vi "_IP Reporter.vi"(4 "ignore Gateway IP?(T)":bool=TRUE, 8 "error in":errorcluster, 9 "notifier":refnum<notifier>, 10 "Init-Information":string, 11 "Setttings":T1={"address"="234.5.6.7", "receiver port"=58432, "Ignore Gateway IP"=TRUE, "HostName"=""}) -> (0 "error out":errorcluster)   [LabVIEW 2017]
doc: "Creates a write-only UDP multicast session and sends data to the specified port."
uses:
  _Typedef/Def-IniSettings -- Cluster.ctl
  _Typedef/Def-Report -- Cluster.ctl
  <vilib>/Utility/tcp.llb/UDP Multicast Write-Only Open.vi
panel:
  out "JSON string":string
  in  "Stop":bool
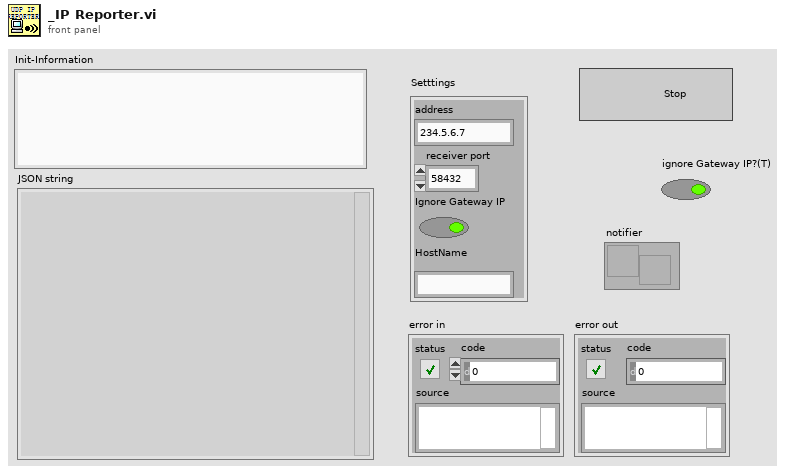
[diagram p1: front panel]
types:
  T1 = typedef "Def-IniSettings -- Cluster.ctl" = cluster{"address":string, "receiver port":u16, "Ignore Gateway IP":bool, "HostName":string}
  T2 = typedef "Def-Report -- Cluster.ctl" = cluster{"Host Name":string, "IPs":string[], "Timestamp":string, "Information":string}
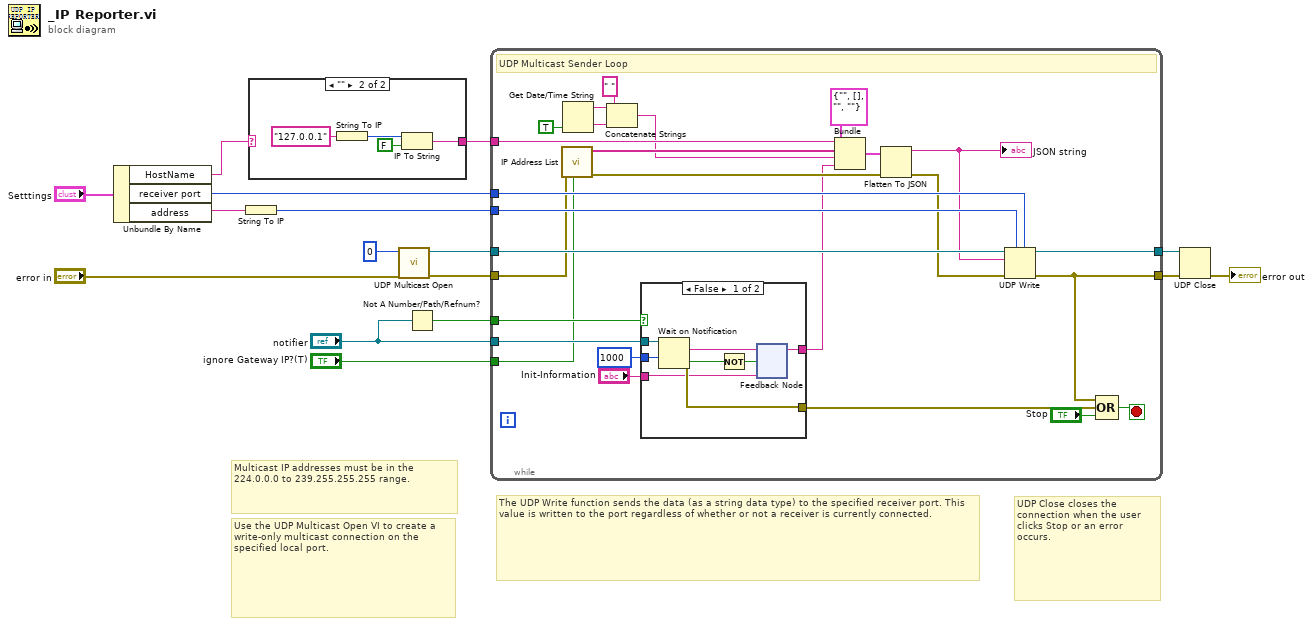
[diagram p0: block diagram]
diagram:
  # "UDP Close closes the connection when the user clicks Stop or an error occurs."
  # "Multicast IP addresses must be in the 224.0.0.0 to 239.255.255.255 range."
  # "The UDP Write function sends the data (as a string data type) to the specified receiver port. This value is written to the port regardless of whether or not a receiver is currently connected."
  # "Use the UDP Multicast Open VI to create a write-only multicast connection on the specified local port."
  n1 = Unbundle By Name("Setttings") -> ("HostName"=w8:string, "receiver port"=w10:u16, "address"=w11:string)
  n2 = String To IP(1:w11) -> (0:w14:u32)
  n3 = case shown="\"\"" w8 {
    selector: w8 -> [w17 _]
    tunnel: [w17 w21] -> w9
    frame "False", Default {
    }
    frame "" {
      n4 = String To IP(1:"127.0.0.1" ("name")) -> (0:w20:u32)
      n5 = IP To String(1:FALSE ("dot notation? (F)"), 2:w20) -> (0:w21:string)
    }
  }
  n6 = call-poly <vilib>:"UDP Multicast Open.vi"("error in (no error)"="error in", "port"=u16 0) -> ("error out"=w12:errorcluster, "connection ID"=w13:refnum<k16>)  [unwired: 8 in]
  n7 = Not A Number/Path/Refnum?(number/path/refnum="notifier") -> (NaN/Path/Refnum?=w6:bool)
  n8 = while {
    tunnel: [w30] -> w15
    tunnel: w13 -> [w48]
    tunnel: w12 -> [w42]
    tunnel: [w45] -> w16
    tunnel: w14 -> [w44]
    tunnel: w10 -> [w43]
    tunnel: w9 -> [w35]
    tunnel: "notifier" -> [w34]
    tunnel: w6 -> [w31]
    tunnel: "ignore Gateway IP?(T)" -> [w24]
    stop <- w47 stop-if-true
    # "UDP Multicast Sender Loop"
    n9 = call "IP Address List.vi"("ignore Gateway IP?"=w24, "error in (no error)"=w42) -> ("error out"=w41:errorcluster, "Array"=w37:string[])  [unwired: 8 in]
    n10 = Get Date/Time String(want seconds? (F)=TRUE) -> (date string=w29:string, time string=w28:string)  [unwired: 2 in]
    n11 = Concatenate Strings(w29, " " ("string"), w28) -> (w26:string)
    n12 = case shown="False" w31 {
      tunnel: w34 -> [w56 _]
      tunnel: 1000 ("timeout in ms (-1)") -> [w55 _]
      tunnel: [w54 _] -> w32
      tunnel: [w50 w57] -> w23
      tunnel: "Init-Information" -> [w49 w57]
      frame False {
        n13 = Wait on Notification(notifier=w56, timeout in ms (-1)=w55) -> (notification=w52:string, timed out?=w53:bool, error out=w54:errorcluster)  [unwired: 2 in, 1 out]
        n14 = Not(x=w53) -> (.not. x?=w51:bool)
        n15 = feedback-in #1(w52, w51) -> ()
        n16 = feedback #1(w49) -> (w50:string)
      }
      frame True {
      }
    }
    n17 = Bundle(cluster=T2 {"Host Name"="", "IPs"=[], "Timestamp"="", "Information"=""} ("Pack"), "Host Name"=w35, "IPs"=w37, "Timestamp"=w26, "Information"=w23) -> (w36:T2)
    n18 = Flatten To JSON(anything=w36, error in (no error)=w41) -> (JSON string=w39:string, 11:w40:errorcluster)  [unwired: 1 in]
    "JSON string" <- w39
    n19 = UDP Write(address=w44, port or service name=w43, connection ID=w48, data in=w39, 8:w40) -> (error out=w30:errorcluster, 3:w45:refnum<k16>)  [unwired: 1 in]
    n20 = Compound Arithmetic op=OR(w30, w32, "Stop") -> (w47:bool)
  }
  n21 = UDP Close(connection ID=w16, 8:w15) -> (error out=→"error out":errorcluster)  [unwired: 1 out]
